vi "Flow Device (Set).vi"(6 "ISOBUS address":T4=-1 caption="ISOBUS address (-1)", 8 "error in":errorcluster, 10 "Heater Device Settings":T3, 11 "Mercury Reference In":T5) -> (0 "error out":errorcluster, 2 "Response":T1, 3 "Mercury Reference Out":T5, 4 "Valid?":T2)   [LabVIEW 2019, in "Mercury iXX.lvlib" / "Flow.lvlib"]
doc: "Set the flow device configuration."
uses:
  Flow.lvlib
  Controls/Mercury Reference.ctl
  CryoTUM_20210311/sub_vi-s/Equipment/Mercury iXX/Public/Controls/Comms Transport Layer.ctl
  Private/Controls/Query Dynamic Reference.ctl
  Controls/ISOBus Address.ctl
  Controls/Flow Device (Set).ctl
  Controls/Is Valid LED.ctl
  Controls/Response String.ctl
  Private/Controls/Command Verbs.ctl
  mercury/Mercury iXX.lvlib
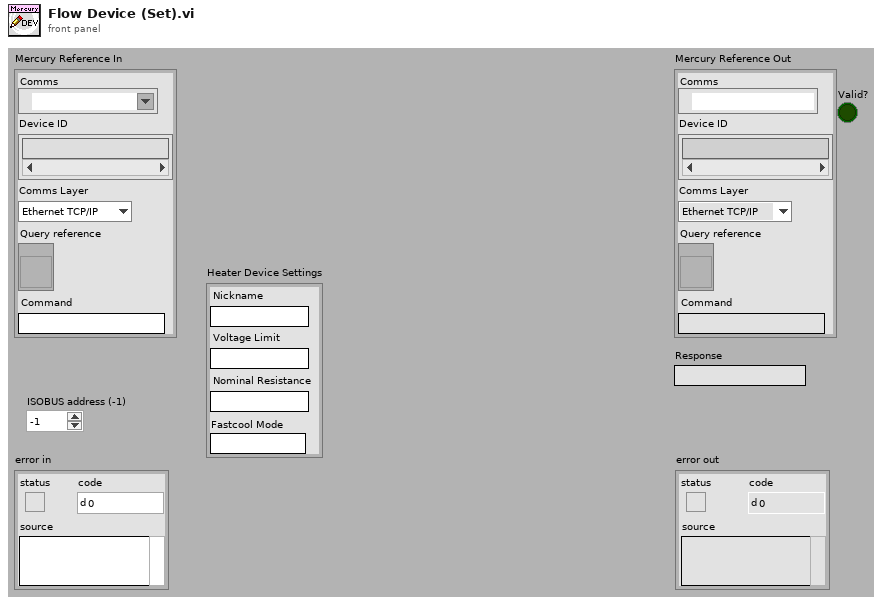
[diagram p1: front panel]
types:
  T1 = typedef "Mercury iXX.lvlib/Response String.ctl" = string
  T2 = typedef "Mercury iXX.lvlib/Is Valid LED.ctl" = bool
  T3 = typedef "Mercury iXX.lvlib/Flow.lvlib/Flow Device (Set).ctl" = cluster{"Nickname":string, "Voltage Limit":string, "Nominal Resistance":string, "Fastcool Mode":string}
  T4 = typedef "Mercury iXX.lvlib/ISOBus Address.ctl" = i32
  T5 = typedef "Mercury iXX.lvlib/Mercury Reference.ctl" = cluster{"Comms":refnum<visa-resource-name>, "Device ID":string[], "Comms Layer":T6, "Command":string, "Query reference":T7}
  T6 = typedef "Mercury iXX.lvlib/Comms Transport Layer.ctl" = enum16{"Ethernet TCP/IP", "USB", "ISOBus - RS-232", "GPIB"}
  T7 = typedef "Mercury iXX.lvlib/Query Dynamic Reference.ctl" = refnum<vi>
  T8 = typedef "Mercury iXX.lvlib/Command Verbs.ctl" = string
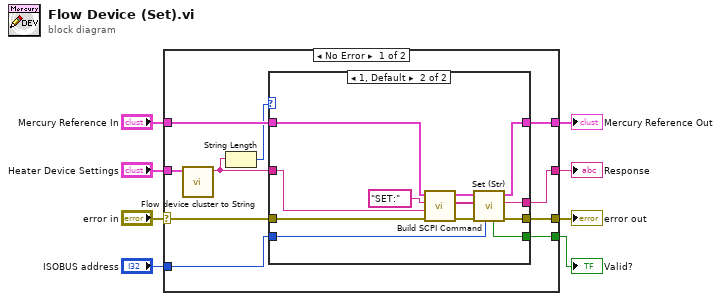
[diagram p0: block diagram]
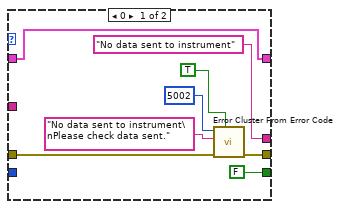
[diagram p2: hidden frame]
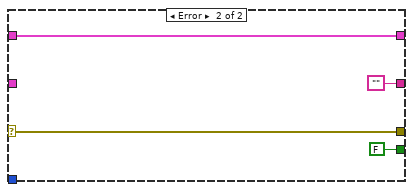
[diagram p3: hidden frame]
diagram:
  n1 = case shown="No Error" "error in" {
    selector: "error in" -> [w17 w41]
    tunnel: "Mercury Reference In" -> [w13 w42]
    tunnel: [w14 w42] -> w7
    tunnel: [w15 w41] -> w6
    tunnel: "ISOBUS address" -> [w16 _]
    tunnel: [w10 ""] -> w2
    tunnel: [w9 FALSE ("Valid?")] -> w3
    tunnel: "Heater Device Settings" -> [w18 _]
    frame No Error {
      n2 = call "Flow device cluster to String.vi"("Heater Device Settings"=w18) -> ("Data to send"=w11:string)  [unwired: 1 in, 9 out]
      n3 = String Length(string=w11) -> (length=w12:i32)
      n4 = case shown="1, Default" w12 {
        tunnel: w13 -> [w26 w32]
        tunnel: w16 -> [_ w28]
        tunnel: w17 -> [w24 w33]
        tunnel: [w25 w34] -> w15
        tunnel: [w26 w31] -> w14
        tunnel: w11 -> [_ w27]
        tunnel: ["No data sent to instrument" ("Data") w30] -> w10
        tunnel: [FALSE ("Valid?") w29] -> w9
        frame 0 {
          n5 = call <vilib>:"Error Cluster From Error Code.vi"("show call chain? (False)"=TRUE, "error in (no error)"=w24, "error message (\"\")"="No data sent to instrument\nPlease check data sent." ("error message (\"\")"), "error code (0)"=5002) -> ("error out"=w25:errorcluster)  [unwired: 5 out]
        }
        frame 1, Default {
          n6 = call "Build SCPI Command.vi"("error in"=w33, "Noun(s)"=w27, "Verb"=T8 "SET:", "Mercury Reference In"=w32) -> ("error out"=w38:errorcluster, "SCPI Message(s)"=w37:string[], "Mercury Reference Out"=w36:T5)  [unwired: 5 out]
          n7 = call "Set (Str).vi"("ISOBUS address"=w28, "error in"=w38, "SCPI Message(s)"=w37, "Mercury Reference In"=w36) -> ("error out"=w34:errorcluster, "Response"=w30:T1, "Mercury Reference Out"=w31:T5, "Valid?"=w29:T2)  [unwired: 1 in, 3 out]
        }
      }
    }
    frame Error {
    }
  }
  "Mercury Reference Out" <- w7
  "error out" <- w6
  "Valid?" <- w3
  "Response" <- w2
